vi "Initialize Obj.vi"(5 "Device":string, 7 "ChanName":string, 8 "error in (no error)":errorcluster, 9 "Timing Engine":T1, 11 "MeasType":T2) -> (0 "error out":errorcluster, 3 "Channel out":refnum<class "Channel.lvclass">)   [LabVIEW 2018, in "Measurement Channels.lvlib" / "Channel.lvclass"]
uses:
  Channel.lvclass
  Custom Ctrls/ge_MeasType.ctl
  Common/Controls/TE_Designator.ctl
  Class Voltage/Voltage.lvclass
  C:/Users/Jeff Tipps/Documents/DAQMan/source/Classes/Measurements/Class Channel/Channel.lvclass
  Class Frequency/Frequency.lvclass
  Class Tachometer/Tachometer.lvclass
  Class Dynamic/Dynamic.lvclass
  Class Thermocouple/Thermocouple.lvclass
  Class RTD/RTD.lvclass
  Class Strain/Strain.lvclass
  Class Current/Current.lvclass
  Class Ressistance/Resistance.lvclass
  Write ChanName.vi
  Write Alias.vi
  Write ModbusAddr.vi
  Write Device.vi
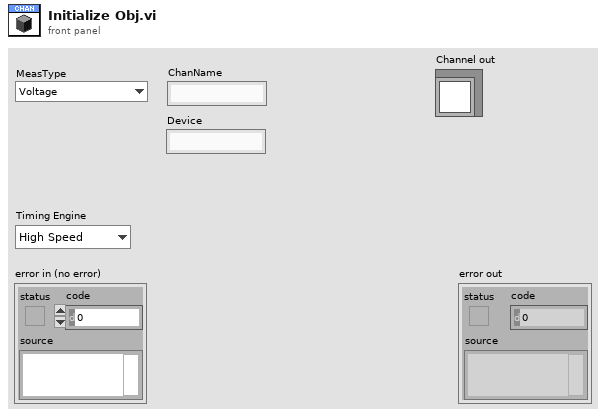
[diagram p1: front panel]
types:
  T1 = typedef "TE_Designator.ctl" = enum16{"High Speed", "Low Speed"}
  T2 = typedef "ge_MeasType.ctl" = enum16{"Voltage", "Frequency", "Tachometer", "Dynamic", "Thermocouple", "RTD", "Strain", "Current", "Resistance"}
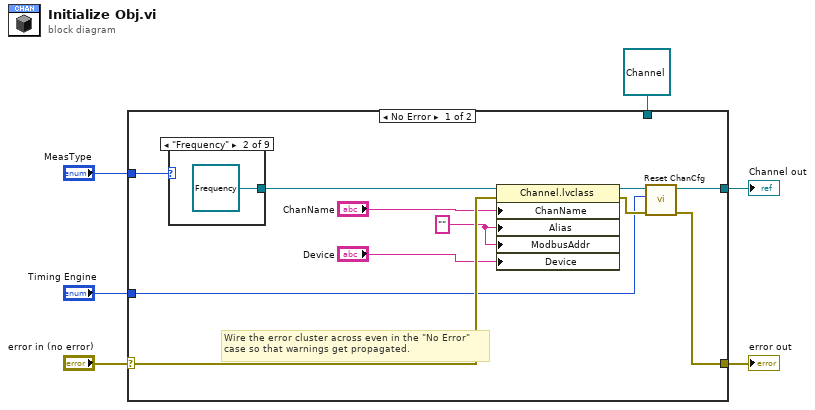
[diagram p0: block diagram]
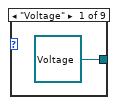
[diagram p2: hidden frame]
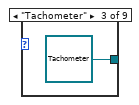
[diagram p3: hidden frame]
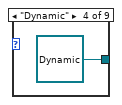
[diagram p4: hidden frame]
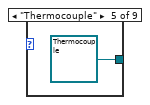
[diagram p5: hidden frame]
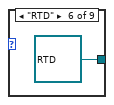
[diagram p6: hidden frame]
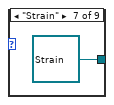
[diagram p7: hidden frame]
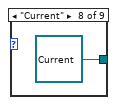
[diagram p8: hidden frame]
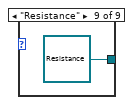
[diagram p9: hidden frame]
diagram:
  n1 = case shown="No Error" "error in (no error)" {
    selector: "error in (no error)" -> [w16 w28]
    tunnel: [w9 w28] -> w5
    tunnel: [w10 w27] -> w4
    tunnel: "MeasType" -> [w17 _]
    tunnel: refnum<class "Channel.lvclass"> refnum ("Dynamic.lvclass") -> [_ w27]
    tunnel: "Timing Engine" -> [w7 _]
    frame No Error {
      w13 = "" ("Alias")
      # "Wire the error cluster across even in the \"No Error\"\ncase so that warnings get propagated."
      n2 = case shown="\"Frequency\"" w17 {
        tunnel: [refnum<class "Voltage.lvclass"> refnum ("Voltage.lvclass") refnum<class "Frequency.lvclass"> refnum ("Frequency.lvclass") refnum<class "Tachometer.lvclass"> refnum ("Tachometer.lvclass") refnum<class "Dynamic.lvclass"> refnum ("Dynamic.lvclass") refnum<class "Thermocouple.lvclass"> refnum ("Thermocouple.lvclass") refnum<class "RTD.lvclass"> refnum ("RTD.lvclass") refnum<class "Strain.lvclass"> refnum ("Strain.lvclass") refnum<class "Current.lvclass"> refnum ("Current.lvclass") refnum<class "Resistance.lvclass"> refnum ("Resistance.lvclass")] -> w12
        frame "Voltage" {
        }
        frame "Frequency" {
        }
        frame "Tachometer" {
        }
        frame "Dynamic" {
        }
        frame "Thermocouple" {
        }
        frame "RTD" {
        }
        frame "Strain" {
        }
        frame "Current" {
        }
        frame "Resistance" {
        }
      }
      n3 = property class="Channel.lvclass"(reference=w12, error in=w16, "ChanName"="ChanName", "Alias"=w13, "ModbusAddr"=w13, "Device"="Device") -> (reference out=w11:refnum<class "Channel.lvclass">, error out=w8:errorcluster)
      n4 = call "Reset ChanCfg.vi"("error in (no error)"=w8, "Timing Engine"=w7, "Channel in"=w11) -> ("error out"=w9:errorcluster, "Channel out"=w10:refnum<class "Channel.lvclass">)  [unwired: 7 in]
    }
    frame Error {
    }
  }
  "error out" <- w5
  "Channel out" <- w4
